vi "getStatusString.vi"(8 "error in (no error)":errorcluster, 11 "Task Status in":refnum<class "Task Status.lvclass">) -> (0 "error out":errorcluster, 2 "Status String":string, 3 "Task Status out":refnum<class "Task Status.lvclass">)   [LabVIEW 2017, in "Message Interface.lvlib" / "Task Status.lvclass"]
uses:
  Task Status.lvclass
  C:/Users/Public/Documents/wc/BuildFarm/src/LabVIEW/vi.lib/BenjaminR/Build Farm/Classes/Message Interface/Status/Status.lvclass
  Status/Status.lvclass/Status.ctl
  Status/Read Status.vi
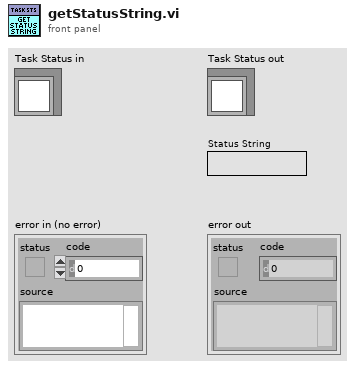
[diagram p1: front panel]
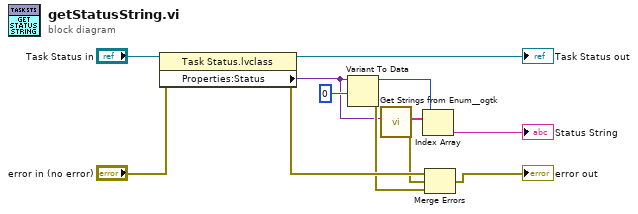
[diagram p0: block diagram]
diagram:
  n1 = property class="Task Status.lvclass"(reference="Task Status in", error in="error in (no error)") -> (reference out=→"Task Status out":refnum<class "Task Status.lvclass">, error out=w5:errorcluster, "Properties:Status"=w1:variant)
  n2 = Variant To Data(type=u16 0, Variant=w1) -> (data=w10:u16, error out=w2:errorcluster)  [unwired: 1 in]
  n3 = call <userlib>:"Get Strings from Enum__ogtk.vi"("Enum"=w1) -> ("error out"=w3:errorcluster, "Enum Strings"=w11:string[])  [unwired: 7 in, 2 out]
  n4 = Index Array(array=w11, index=w10) -> (element=→"Status String":string)
  n5 = Merge Errors(w5, w3, w2) -> (→"error out":errorcluster)
